vi "szyfr.vi"(8 "Numeric":dbl, 11 "String":string) -> (2 "String 2":string)   [LabVIEW 2022 SP3]
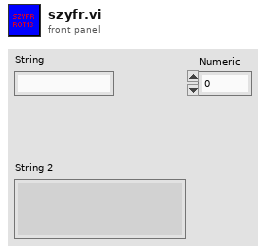
[diagram p1: front panel]
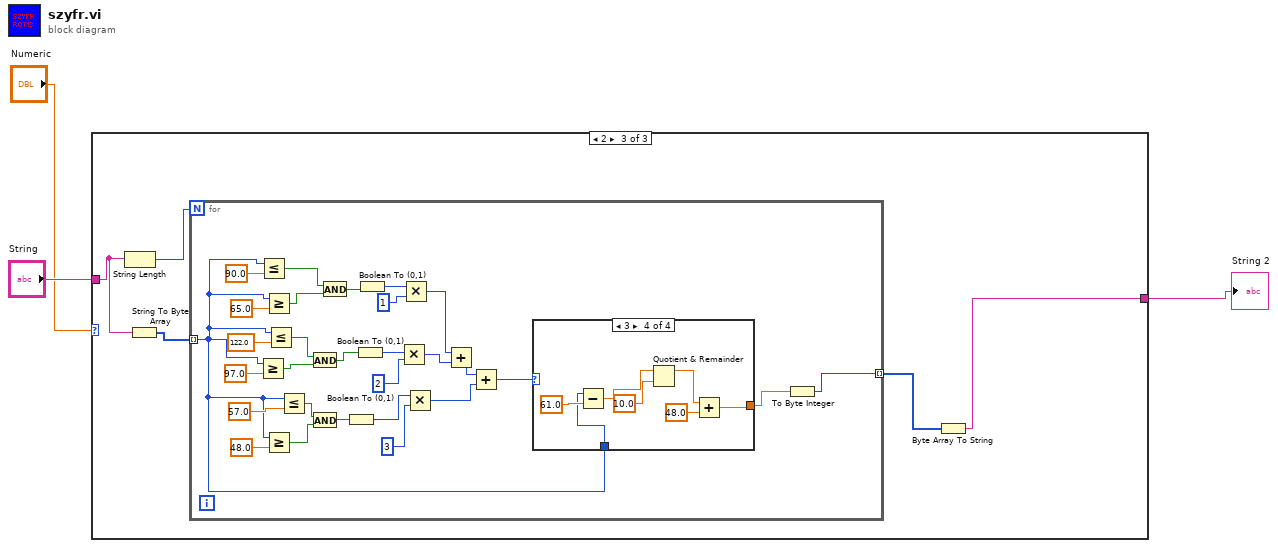
[diagram p0: block diagram]
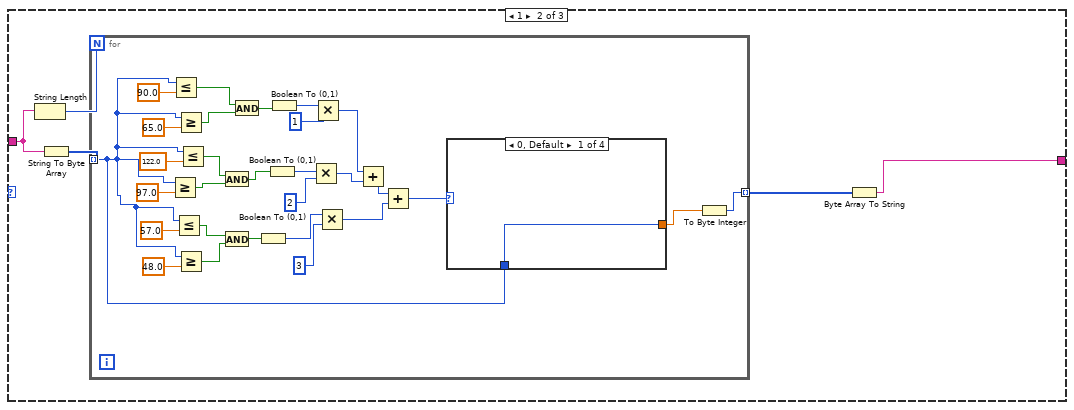
[diagram p3: hidden frame]
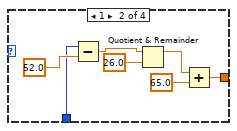
[diagram p4: hidden frame]
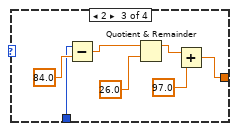
[diagram p5: hidden frame]
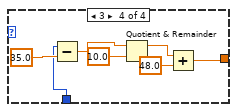
[diagram p6: hidden frame]
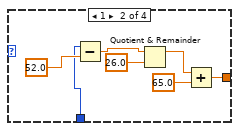
[diagram p8: hidden frame]
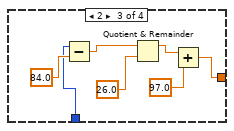
[diagram p9: hidden frame]
diagram:
  n1 = case shown="2" "Numeric" {
    tunnel: "String" -> [w4 w8 w64]
    tunnel: [w4 w6 w61] -> w1
    frame 0, Default {
    }
    frame 1 {
      n2 = String Length(string=w8) -> (length=w9:i32)
      n3 = String To Byte Array(string=w8) -> (unsigned byte array=w7:u8[])
      n4 = for {
        N: w9 -> [_]
        tunnel: w7 -> [w10] mode=indexing
        tunnel: [w11] -> w5 mode=indexing
        n5 = Greater Or Equal?(x=w10, y=97.0) -> (x >= y?=w31:bool)
        n6 = Less Or Equal?(x=w10, y=90.0) -> (x <= y?=w35:bool)
        n7 = Less Or Equal?(x=w10, y=57.0) -> (x <= y?=w28:bool)
        n8 = Greater Or Equal?(x=w10, y=65.0) -> (x >= y?=w36:bool)
        n9 = Greater Or Equal?(x=w10, y=48.0) -> (x >= y?=w27:bool)
        n10 = Less Or Equal?(x=w10, y=122.0) -> (x <= y?=w32:bool)
        n11 = And(x=w32, y=w31) -> (x .and. y?=w25:bool)
        n12 = And(x=w28, y=w27) -> (x .and. y?=w24:bool)
        n13 = And(x=w35, y=w36) -> (x .and. y?=w26:bool)
        n14 = Boolean To (0,1)(Boolean=w24) -> (0, 1=w21:i16)
        n15 = Boolean To (0,1)(Boolean=w25) -> (0, 1=w22:i16)
        n16 = Boolean To (0,1)(Boolean=w26) -> (0, 1=w23:i16)
        n17 = Multiply(x=w22, y=i16 2) -> (x*y=w16:i16)
        n18 = Multiply(x=w23, y=i16 1) -> (x*y=w17:i16)
        n19 = Multiply(x=w21, y=i16 3) -> (x*y=w14:i16)
        n20 = Add(x=w17, y=w16) -> (x+y=w15:i16)
        n21 = Add(x=w15, y=w14) -> (x+y=w13:i16)
        n22 = case shown="0, Default" w13 {
          tunnel: [w39 w41 w48 w55] -> w12
          tunnel: w10 -> [w39 w40 w47 w54]
          frame 0, Default {
          }
          frame 1 {
            n23 = Subtract(x=w40, y=52.0) -> (x-y=w44:dbl)
            n24 = Quotient & Remainder(x=w44, y=26.0) -> (x-y*floor(x/y)=w42:dbl)  [unwired: 1 out]
            n25 = Add(x=w42, y=65.0) -> (x+y=w41:dbl)
          }
          frame 2 {
            n26 = Subtract(x=w47, y=84.0) -> (x-y=w52:dbl)
            n27 = Quotient & Remainder(x=w52, y=26.0) -> (x-y*floor(x/y)=w49:dbl)  [unwired: 1 out]
            n28 = Add(x=w49, y=97.0) -> (x+y=w48:dbl)
          }
          frame 3 {
            n29 = Subtract(x=w54, y=35.0) -> (x-y=w58:dbl)
            n30 = Quotient & Remainder(x=w58, y=10.0) -> (x-y*floor(x/y)=w56:dbl)  [unwired: 1 out]
            n31 = Add(x=w56, y=48.0) -> (x+y=w55:dbl)
          }
        }
        n32 = To Byte Integer(number=w12) -> (8bit integer=w11:i8)
      }
      n33 = Byte Array To String(unsigned byte array=w5) -> (string=w6:string)
    }
    frame 2 {
      n34 = String Length(string=w64) -> (length=w63:i32)
      n35 = String To Byte Array(string=w64) -> (unsigned byte array=w62:u8[])
      n36 = for {
        N: w63 -> [_]
        tunnel: [w67] -> w65 mode=indexing
        tunnel: w62 -> [w66] mode=indexing
        n37 = Greater Or Equal?(x=w66, y=97.0) -> (x >= y?=w80:bool)
        n38 = Less Or Equal?(x=w66, y=90.0) -> (x <= y?=w78:bool)
        n39 = Greater Or Equal?(x=w66, y=65.0) -> (x >= y?=w77:bool)
        n40 = Greater Or Equal?(x=w66, y=48.0) -> (x >= y?=w82:bool)
        n41 = Less Or Equal?(x=w66, y=122.0) -> (x <= y?=w79:bool)
        n42 = Less Or Equal?(x=w66, y=57.0) -> (x <= y?=w81:bool)
        n43 = And(x=w79, y=w80) -> (x .and. y?=w84:bool)
        n44 = And(x=w81, y=w82) -> (x .and. y?=w85:bool)
        n45 = And(x=w78, y=w77) -> (x .and. y?=w83:bool)
        n46 = Boolean To (0,1)(Boolean=w85) -> (0, 1=w88:i16)
        n47 = Boolean To (0,1)(Boolean=w84) -> (0, 1=w87:i16)
        n48 = Boolean To (0,1)(Boolean=w83) -> (0, 1=w86:i16)
        n49 = Multiply(x=w87, y=i16 2) -> (x*y=w90:i16)
        n50 = Multiply(x=w86, y=i16 1) -> (x*y=w89:i16)
        n51 = Multiply(x=w88, y=i16 3) -> (x*y=w92:i16)
        n52 = Add(x=w89, y=w90) -> (x+y=w91:i16)
        n53 = Add(x=w91, y=w92) -> (x+y=w93:i16)
        n54 = case shown="3" w93 {
          tunnel: [w95 w97 w104 w111] -> w94
          tunnel: w66 -> [w95 w96 w103 w110]
          frame 0, Default {
          }
          frame 1 {
            n55 = Subtract(x=w96, y=52.0) -> (x-y=w100:dbl)
            n56 = Quotient & Remainder(x=w100, y=26.0) -> (x-y*floor(x/y)=w98:dbl)  [unwired: 1 out]
            n57 = Add(x=w98, y=65.0) -> (x+y=w97:dbl)
          }
          frame 2 {
            n58 = Subtract(x=w103, y=84.0) -> (x-y=w108:dbl)
            n59 = Quotient & Remainder(x=w108, y=26.0) -> (x-y*floor(x/y)=w105:dbl)  [unwired: 1 out]
            n60 = Add(x=w105, y=97.0) -> (x+y=w104:dbl)
          }
          frame 3 {
            n61 = Subtract(x=w110, y=61.0) -> (x-y=w114:dbl)
            n62 = Quotient & Remainder(x=w114, y=10.0) -> (x-y*floor(x/y)=w112:dbl)  [unwired: 1 out]
            n63 = Add(x=w112, y=48.0) -> (x+y=w111:dbl)
          }
        }
        n64 = To Byte Integer(number=w94) -> (8bit integer=w67:i8)
      }
      n65 = Byte Array To String(unsigned byte array=w65) -> (string=w61:string)
    }
  }
  "String 2" <- w1
